vi "20210714_SR400 monitoring_sub.vi"(7 "VISA resource name":refnum<visa-resource-name>="GPIB0::18::INSTR", 8 "DigNum Refnum":refnum<vi>, 9 "Ctl Refnum":refnum<vi>, 10 "stop Refnum":refnum<vi>, 11 "?":bool) -> ()   [LabVIEW 2015]
uses:
  Libraries/SR400/Public/Typedefs/Counter.ctl
  Libraries/SR400/SR400.lvlib
panel:
  in  "Count Time Set":dbl[unit]=0.01
  out "Count plot":dbl(graph)=137.0
  out "Counts":dbl format="%#_6e"
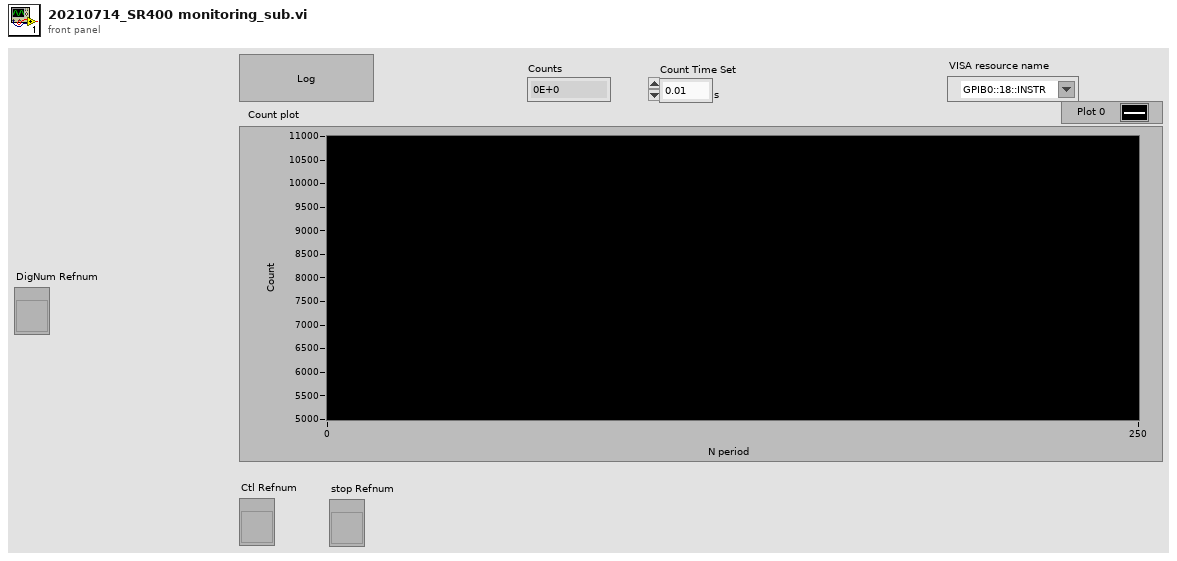
[diagram p1: front panel]
types:
  T1 = enum16{"open", "replace", "create", "open or create", "replace or create", "replace or create with confirmation"}
  T2 = typedef "SR400.lvlib/Counter.ctl" = enum16{"Counter A", "Counter B", "Counter T"}
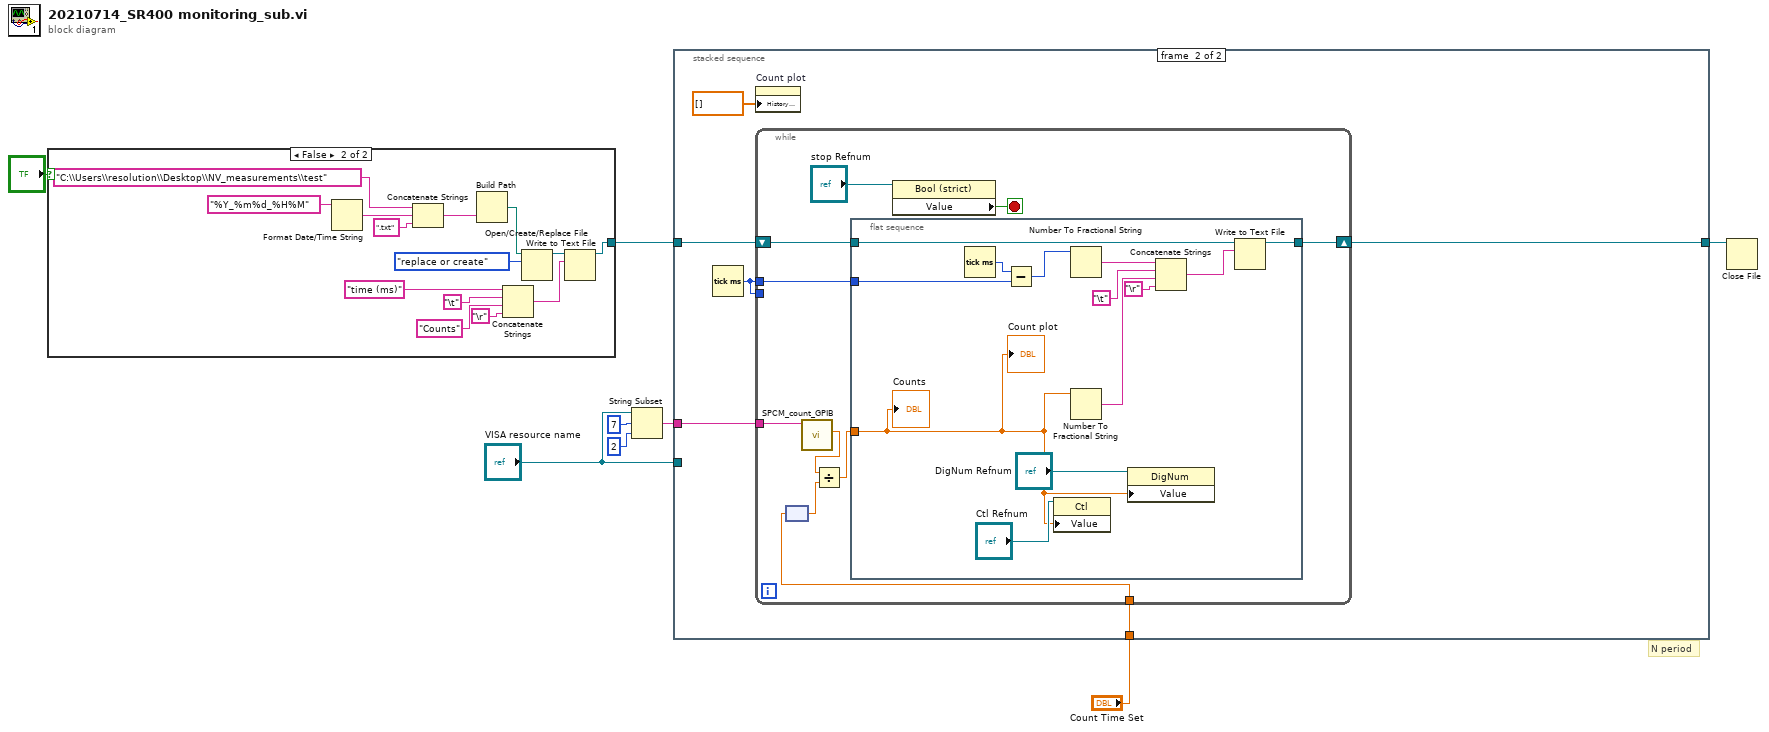
[diagram p0: block diagram]
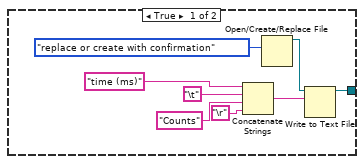
[diagram p2: hidden frame]
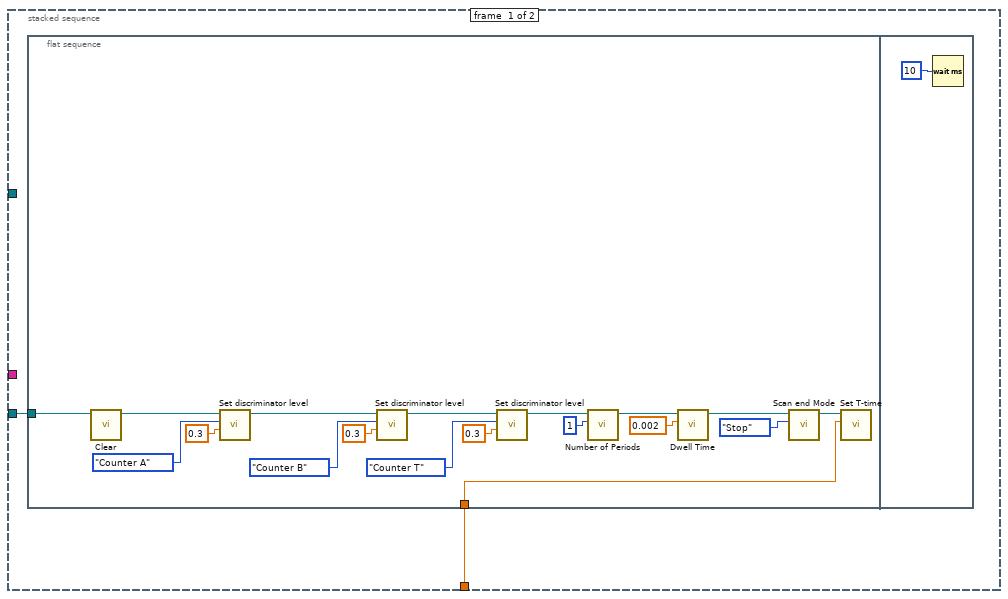
[diagram p3: hidden frame]
diagram:
  # "N period"
  n1 = case shown="False" "?" {
    tunnel: [w9 w22] -> w7
    frame True {
      n2 = Concatenate Strings("time (ms)" ("string"), "\t", "Counts" ("string"), "\r") -> (w15:string)
      n3 = Open/Create/Replace File(operation (0:open)=T1."replace or create with confirmation") -> (refnum out=w16:refnum<file>)  [unwired: 5 in, 2 out]
      n4 = Write to Text File(file (use dialog)=w16, text=w15) -> (refnum out=w9:refnum<file>)  [unwired: 2 in, 2 out]
    }
    frame False {
      n5 = Format Date/Time String(time format string (%c)="%Y_%m%d_%H%M") -> (date/time string=w27:string)  [unwired: 2 in]
      n6 = Concatenate Strings("C:\\Users\\resolution\\Desktop\\NV_measurements\\test" ("string"), w27, ".txt" ("string")) -> (w26:string)
      n7 = Build Path(name or relative path=w26) -> (appended path=w30:path)  [unwired: 1 in]
      n8 = Concatenate Strings("time (ms)" ("string"), "\t", "Counts" ("string"), "\r") -> (w17:string)
      n9 = Open/Create/Replace File(file path (use dialog)=w30, operation (0:open)=T1."replace or create") -> (refnum out=w23:refnum<file>)  [unwired: 4 in, 2 out]
      n10 = Write to Text File(file (use dialog)=w23, text=w17) -> (refnum out=w22:refnum<file>)  [unwired: 2 in, 2 out]
    }
  }
  n11 = String Subset(string="VISA resource name", offset (0)=7, length (rest)=2 ("length (rest)")) -> (substring=w2:string)
  n12 = stacked-sequence {
    tunnel: w2 -> [_ w57]
    tunnel: w7 -> [_ w55]
    tunnel: [_ w54] -> w6
    tunnel: "VISA resource name" -> [w32 _]
    tunnel: "Count Time Set" -> [w31 w52]
    frame #0 {
      n13 = flat-sequence {
        tunnel: w32 -> [w35]
        tunnel: w31 -> [w33]
        frame #0 {
          n14 = call "Clear.vi"("VISA resource name"=w35) -> ("VISA resource name out"=w50:refnum<visa-resource-name>)  [unwired: 9 in, 1 out]
          n15 = call "Set discriminator level.vi"("Level (-0.034 V)"=0.3, "Discriminator (def: A)"=Counter."Counter A", "VISA resource name"=w50) -> ("VISA resource name out"=w47:refnum<visa-resource-name>)  [unwired: 7 in, 1 out]
          n16 = call "Set discriminator level.vi"("Level (-0.034 V)"=0.3, "Discriminator (def: A)"=Counter."Counter B", "VISA resource name"=w47) -> ("VISA resource name out"=w44:refnum<visa-resource-name>)  [unwired: 7 in, 1 out]
          n17 = call "Set discriminator level.vi"("Level (-0.034 V)"=0.3, "Discriminator (def: A)"=Counter."Counter T", "VISA resource name"=w44) -> ("VISA resource name out"=w41:refnum<visa-resource-name>)  [unwired: 7 in, 1 out]
          n18 = call "Number of Periods.vi"("# of periods (def: 1)"=1, "VISA resource name"=w41) -> ("VISA resource name out"=w39:refnum<visa-resource-name>)  [unwired: 8 in, 1 out]
          n19 = call "Dwell Time.vi"("Dwell time (0.002 s)"=0.002, "VISA resource name"=w39) -> ("VISA resource name out"=w37:refnum<visa-resource-name>)  [unwired: 8 in, 1 out]
          n20 = call "Scan end Mode.vi"("Scan End Mode (Def: Stop)"=enum16{"Stop", "Start"}."Stop", "VISA resource name"=w37) -> ("VISA resource name out"=w34:refnum<visa-resource-name>)  [unwired: 8 in, 1 out]
          n21 = call "Set T-time.vi"("Count Time Set"=w33, "VISA resource name"=w34) -> ()  [unwired: 5 in, 3 out]
        }
        frame #1 {
          n22 = Wait (ms)(milliseconds to wait=u32 10) -> ()  [unwired: 1 out]
        }
      }
    }
    frame #1 {
      n23 = Tick Count (ms)() -> (millisecond timer value=w53:u32)
      n24 = property on="Count plot" class="WFChart (strict)"("History Data"=dbl[] []) -> ()  [unwired: 2 in, 2 out]
      n25 = while {
        tunnel: w57 -> [w67]
        tunnel: w53 -> [_]
        tunnel: w53 -> [w65]
        shift-right: [w64] -> w54
        shift-left: w55 -> [w66]
        tunnel: w52 -> [w61]
        stop <- w62 stop-if-true
        n26 = node(w61) -> (w60:dbl)
        n27 = call "SPCM_count_GPIB.vi"("SR400 GPIB Address"=w67) -> ("Counts"=w59:dbl)  [unwired: 10 in]
        n28 = Divide(x=w59, y=w60) -> (x/y=w58:dbl)
        n29 = flat-sequence {
          tunnel: w58 -> [w68]
          tunnel: w66 -> [w72]
          tunnel: w65 -> [w79]
          tunnel: [w71] -> w64
          frame #0 {
            n30 = Tick Count (ms)() -> (millisecond timer value=w80:u32)
            n31 = Subtract(x=w80, y=w79) -> (x-y=w76:u32)
            n32 = property class="Ctl"(reference="Ctl Refnum", "Value"=w68) -> ()  [unwired: 1 in, 2 out]
            n33 = Number To Fractional String(number=w76) -> (F-format string=w75:string)  [unwired: 3 in]
            n34 = Number To Fractional String(number=w68) -> (F-format string=w74:string)  [unwired: 3 in]
            n35 = property class="DigNum"(reference="DigNum Refnum", "Value"=w68) -> ()  [unwired: 1 in, 2 out]
            n36 = Concatenate Strings(w75, "\t", w74, "\r") -> (w73:string)
            n37 = Write to Text File(file (use dialog)=w72, text=w73) -> (refnum out=w71:refnum<file>)  [unwired: 2 in, 2 out]
            "Count plot" <- w68
            "Counts" <- w68
          }
        }
        n38 = property class="Bool (strict)"(reference="stop Refnum") -> ("Value"=w62:bool)  [unwired: 1 in, 2 out]
      }
    }
  }
  n39 = Close File(refnum=w6) -> ()  [unwired: 1 in, 2 out]
